vi "Steps DAO.vi"(8 "error in (no error)":errorcluster, 9 "Step String In":string, 10 "Step In":i32, 11 "Steps Actions":T2(ring)) -> (0 "error out":errorcluster, 1 "Steps Out":T1, 2 "Step String Out":string)   [LabVIEW 2009]
uses:
  Steps Type.ctl
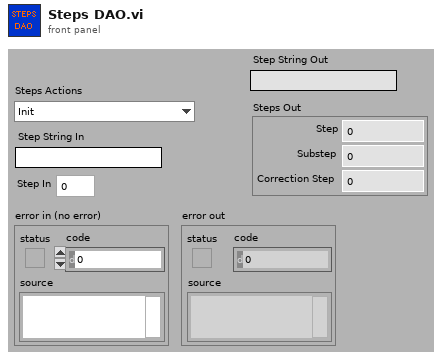
[diagram p1: front panel]
types:
  T1 = typedef "Steps Type.ctl" = cluster{"Step":i32, "Substep":i32, "Correction Step":i32}
  T2 = enum16{"Init", "Set Step", "Set Correction Step", "Set Step String", "Get Step String"}
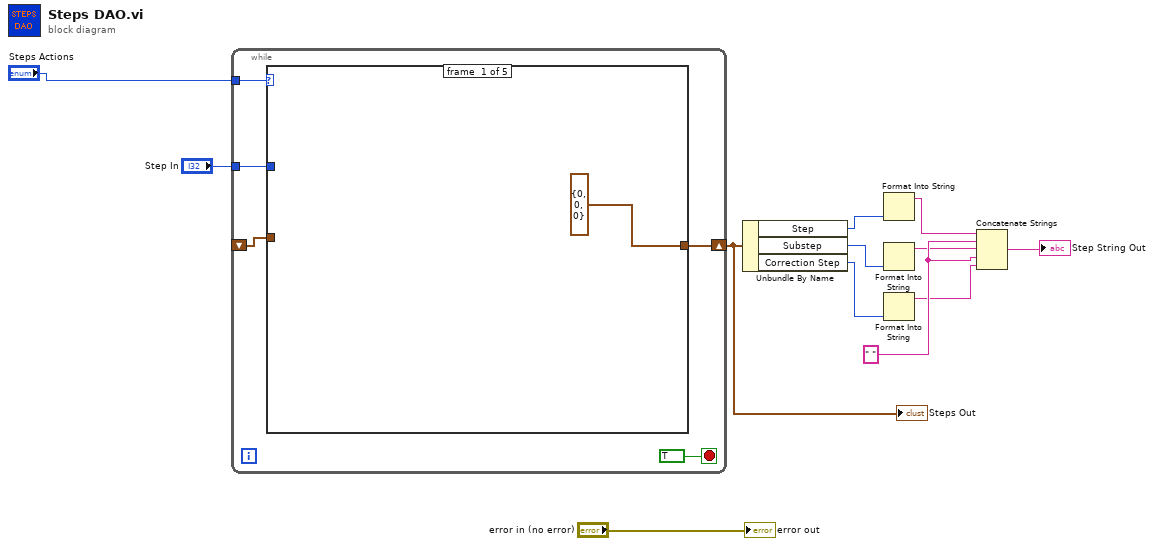
[diagram p0: block diagram]
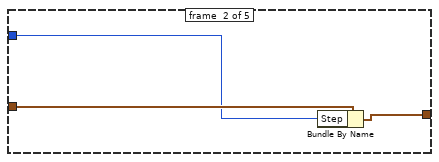
[diagram p2: hidden frame]
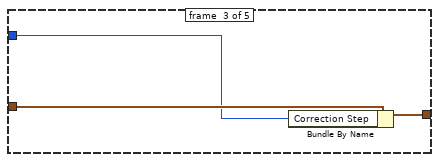
[diagram p3: hidden frame]
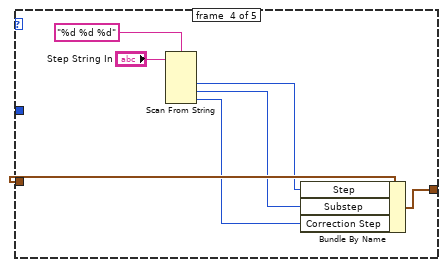
[diagram p4: hidden frame]
diagram:
  w9 = " " ("string")
  n1 = while {
    tunnel: "Steps Actions" -> [w16]
    shift-right: [w15] -> w10
    shift-left: _ -> [w14]
    tunnel: "Step In" -> [w13]
    stop <- TRUE stop-if-true
    n2 = case shown="\"Set Step\"" w16 {
      tunnel: [T1 {"Step"=0, "Substep"=0, "Correction Step"=0} ("Steps") w19 w22 w28 w32] -> w15
      tunnel: w14 -> [_ w21 w24 w29 w32]
      tunnel: w13 -> [_ w20 w23 _ _]
      frame #0 {
      }
      frame #1 {
        n3 = Bundle By Name(cluster=w21, "Step"=w20) -> (w19:T1)
      }
      frame #2 {
        n4 = Bundle By Name(cluster=w24, "Correction Step"=w23) -> (w22:T1)
      }
      frame #3 {
        n5 = Scan From String(format string="%d %d %d", input string="Step String In") -> (output 1=w27:i32, output 2=w26:i32, output 3=w25:i32)  [unwired: 5 in, 3 out]
        n6 = Bundle By Name(cluster=w29, "Step"=w27, "Substep"=w26, "Correction Step"=w25) -> (w28:T1)
      }
      frame #4 {
      }
    }
  }
  "Steps Out" <- w10
  n7 = Unbundle By Name(w10) -> ("Step"=w8:i32, "Substep"=w7:i32, "Correction Step"=w6:i32)
  n8 = Format Into String(w8) -> (resulting string=w5:string)  [unwired: 3 in, 1 out]
  n9 = Format Into String(w7) -> (resulting string=w4:string)  [unwired: 3 in, 1 out]
  n10 = Format Into String(w6) -> (resulting string=w3:string)  [unwired: 3 in, 1 out]
  n11 = Concatenate Strings(w5, w9, w4, w9, w3) -> (→"Step String Out":string)
  "error out" <- "error in (no error)"
